vi "Reset.vi"(8 "error in (no error)":errorcluster, 11 "ClassIn":refnum<class "Keysight335XX.lvclass">) -> (0 "error out":errorcluster, 3 "ClassOut":refnum<class "Keysight335XX.lvclass">)   [LabVIEW 2014, in "FGenPlugins.lvlib" / "Keysight335XX.lvclass"]
uses:
  Keysight335XX.lvclass
  <instrlib>/Agilent 3352X Series/Agilent 3352X Series.lvlib
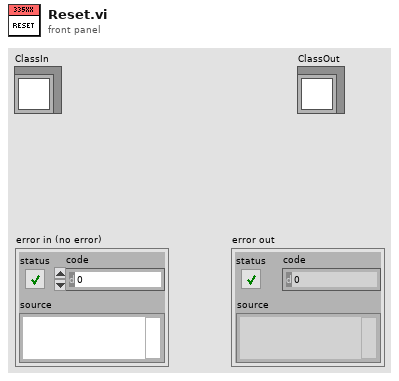
[diagram p1: front panel]
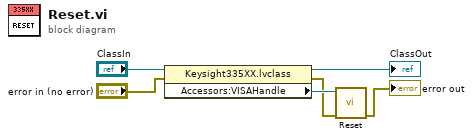
[diagram p0: block diagram]
diagram:
  n1 = property class="Keysight335XX.lvclass"(reference="ClassIn", error in="error in (no error)") -> (reference out=→"ClassOut":refnum<class "Keysight335XX.lvclass">, error out=w5:errorcluster, "Accessors:VISAHandle"=w6:refnum<visa-resource-name>)
  n2 = call <instrlib>:"Reset.vi"("error in (no error)"=w5, "VISA resource name"=w6) -> ("error out"=→"error out":errorcluster)  [unwired: 8 in, 1 out]
